vi "Initialization_IPS120_ver1.0.vi"(0 "Magnet Control (IPS 120-10)":T2={"Action"=1, "Standby (s)"=0.0, "Heater on (s)"=300.0, "Sweep Steps "=[], "GPIB ADR"=0, "Change Para?"=FALSE} {"GPIB ADR" items=["None"=0, "25"=25]; "Sweep Steps"."Hold(min)" min=0.0; "Sweep Steps"."Set Rate(T/min)" min=0.001 max=0.5 step=0.001; "Sweep Steps"."Set Point (T)" min=-9.0 max=9.0 step=0.001; "Action" items=["Hold", "To Set Point", "To Zero", "Clamp"]}, 2 "error in":errorcluster, 4 "First run?":bool) -> (1 "Magnet Failed?":bool, 3 "Hold(min)":dbl, 5 "Status":string, 6 "B field Change?":bool, 7 "output cluster":T1={"Com Port"=1, "ISOBUS Address"=1, "GPIB Address"=24, "Communication"=enum."ISOBUS"}, 8 "Target B":string, 9 "Rate":string, 10 "error out":errorcluster)   [LabVIEW 2012]
uses:
  Oxford_itc503/BUSGEN.LLB/OxfordAddress.ctl
panel:
  out "Set point":string
  out "Display":string="+0.00000\r"
  out "Log":string
  # "Current\nField"
  # "T"
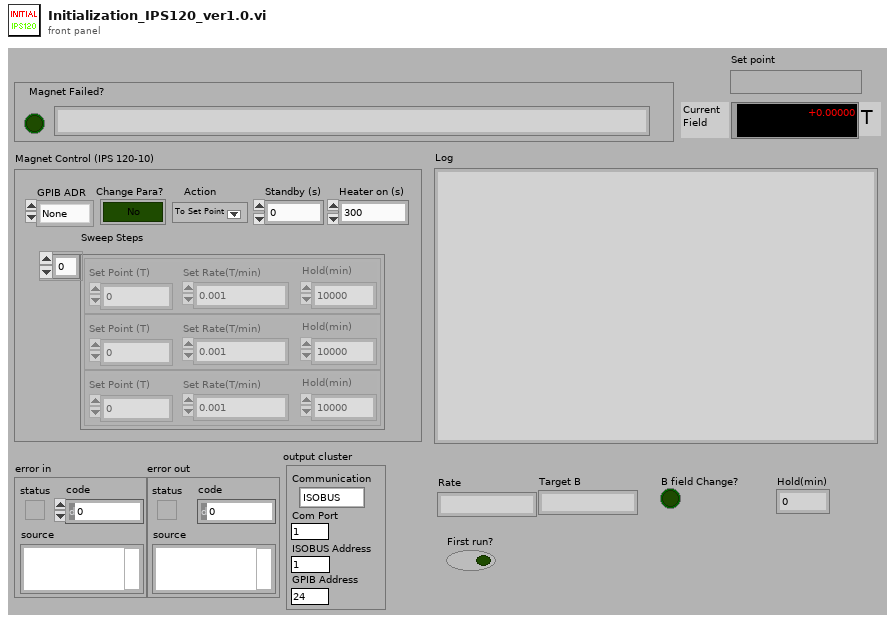
[diagram p1: front panel]
types:
  T1 = cluster{"Com Port":i32, "ISOBUS Address":i32, "GPIB Address":i16, "Communication":enum16{"RS232", "ISOBUS", "GPIB", "Gateway"}}
  T2 = cluster{"Action":u16, "Standby (s)":dbl, "Heater on (s)":dbl, "Sweep Steps ":cluster{"Set Point (T)":dbl, "Set Rate(T/min)":dbl, "Hold(min)":dbl}[], "GPIB ADR":u16, "Change Para?":bool}
  T3 = typedef "OxfordAddress.ctl" = cluster{"Com Port":i32, "ISOBUS Address":i32, "GPIB Address":i16, "Communication":enum16{"RS232", "ISOBUS", "GPIB", "Gateway"}}
  T4 = cluster{"Set Point (T)":dbl, "Set Rate(T/min)":dbl, "Hold(min)":dbl}[]
  T5 = cluster{"Set Point (T)":dbl, "Set Rate(T/min)":dbl, "Hold(min)":dbl}
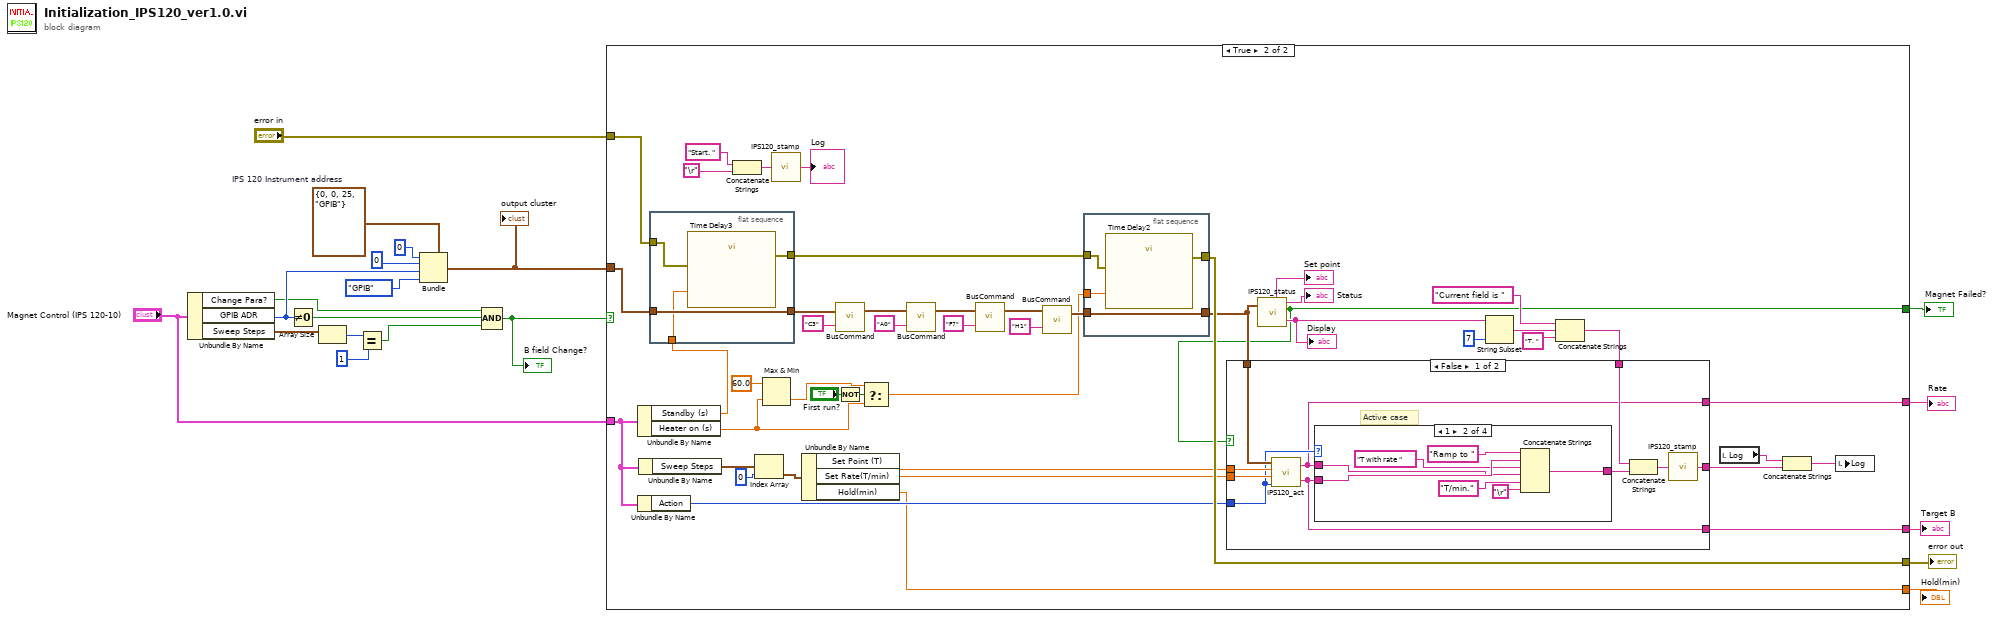
[diagram p0: block diagram]
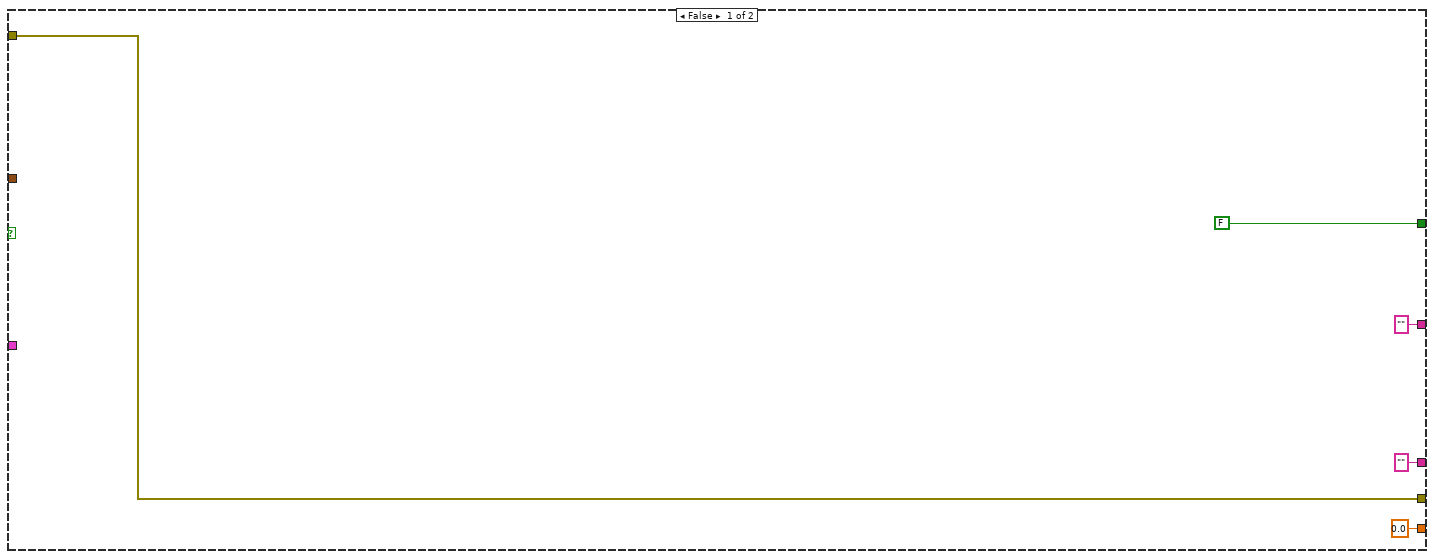
[diagram p2: hidden frame]
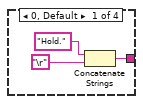
[diagram p3: hidden frame]
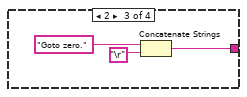
[diagram p4: hidden frame]
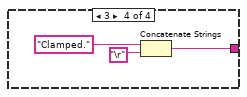
[diagram p5: hidden frame]
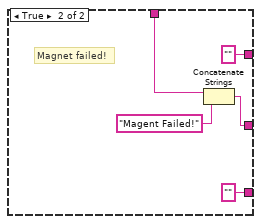
[diagram p6: hidden frame]
diagram:
  w14 = T3 {"Com Port"=0, "ISOBUS Address"=0, "GPIB Address"=25, "Communication"=enum."GPIB"}  # IPS 120 Instrument address
  n1 = Unbundle By Name("Magnet Control (IPS 120-10)") -> ("Change Para?"=w7:bool, "GPIB ADR"=w12:u16, "Sweep Steps"=w11:T4)
  n2 = Not Equal To 0?(x=w12) -> (x != 0?=w6:bool)
  n3 = Array Size(array=w11) -> (size(s)=w10:i32)
  n4 = Equal?(x=w10, y=1) -> (x = y?=w5:bool)
  n5 = Bundle(cluster=w14, "Com Port"=0, "ISOBUS Address"=0, "GPIB Address"=w12, "Communication"=enum16{"RS232", "ISOBUS", "GPIB", "Gateway"}."GPIB") -> (w13:T3)
  "output cluster" <- w13
  n6 = Compound Arithmetic op=AND(w7, w6, w5) -> (w8:bool)
  "B field Change?" <- w8
  n7 = case shown="True" w8 {
    tunnel: "Magnet Control (IPS 120-10)" -> [_ w37]
    tunnel: [w24 w55] -> w19
    tunnel: "error in" -> [w24 w54]
    tunnel: w13 -> [_ w53]
    tunnel: [FALSE w35] -> w4
    tunnel: ["" ("Rate") w34] -> w3
    tunnel: ["" ("Target B") w33] -> w2
    tunnel: [0.0 ("Hold(min)") w32] -> w1
    frame False {
    }
    frame True {
      n8 = Unbundle By Name(w37) -> ("Standby (s)"=w38:dbl, "Heater on (s)"=w28:dbl)
      n9 = Unbundle By Name(w37) -> ("Action"=w36:u16)
      n10 = Unbundle By Name(w37) -> ("Sweep Steps"=w58:T4)
      n11 = flat-sequence {
        tunnel: w53 -> [w107]
        tunnel: [w107] -> w60
        tunnel: w38 -> [w106]
        tunnel: w54 -> [w105]
        tunnel: [w104] -> w59
        frame #0 {
          n12 = call "Time Delay3"("error in (no error)"=w105, "Delay Time (s)"=w106) -> ("error out"=w104:errorcluster)  [unwired: 9 in]
        }
      }
      n13 = Concatenate Strings("Start. " ("Log"), "\r") -> (w70:string)
      n14 = Index Array(array=w58, index=0) -> (element=w56:T5)
      n15 = Max & Min(x=60.0 ("t"), y=w28) -> (min(x,y)=w26:dbl)  [unwired: 1 out]
      n16 = call "IPS120_stamp.vi"("in"=w70) -> ("out"=→"Log":string)
      n17 = Unbundle By Name(w56) -> ("Set Point (T)"=w52:dbl, "Set Rate(T/min)"=w51:dbl, "Hold(min)"=w32:dbl)
      n18 = call "BusCommand.vi"("Command"="C3", "Instrument address (in)"=w60) -> ("Instrument address (out)"=w67:T3)  [unwired: 1 out]
      n19 = Not(x="First run?") -> (.not. x?=w27:bool)
      n20 = Select(t=w26, s=w27, f=w28) -> (s? t:f=w30:dbl)
      n21 = call "BusCommand.vi"("Command"="A0", "Instrument address (in)"=w67) -> ("Instrument address (out)"=w66:T3)  [unwired: 1 out]
      n22 = call "BusCommand.vi"("Command"="F7", "Instrument address (in)"=w66) -> ("Instrument address (out)"=w61:T3)  [unwired: 1 out]
      n23 = call "BusCommand.vi"("Command"="H1", "Instrument address (in)"=w61) -> ("Instrument address (out)"=w62:T3)  [unwired: 1 out]
      n24 = flat-sequence {
        tunnel: w62 -> [w111]
        tunnel: [w111] -> w47
        tunnel: w30 -> [w110]
        tunnel: w59 -> [w109]
        tunnel: [w108] -> w55
        frame #0 {
          n25 = call "Time Delay2"("error in (no error)"=w109, "Delay Time (s)"=w110) -> ("error out"=w108:errorcluster)  [unwired: 9 in]
        }
      }
      n26 = call "IPS120_status.vi"("Address"=w47) -> ("Set point"=→"Set point":string, "Real Field"=w50:string, "Staus"=→"Status":string, "Magnet Failed?"=w35:bool)  [unwired: 1 in, 2 out]
      "Display" <- w50
      n27 = String Subset(string=w50, length (rest)=7 ("length (rest)")) -> (substring=w41:string)  [unwired: 1 in]
      n28 = Concatenate Strings("Current field is " ("string"), w41, "T. " ("string")) -> (w39:string)
      n29 = case shown="False" w35 {
        tunnel: w52 -> [w82 _]
        tunnel: w51 -> [w81 _]
        tunnel: w47 -> [w80 _]
        tunnel: [w79 w101] -> w44
        tunnel: w39 -> [w77 w103]
        tunnel: w36 -> [w75 _]
        tunnel: [w74 "" ("Rate")] -> w34
        tunnel: [w73 "" ("Target B")] -> w33
        frame False {
          # "Active case"
          n30 = call "IPS120_act.vi"("Action"=w75, "Set Rate"=w81, "Set Point"=w82, "Address"=w80) -> ("Target B"=w73:string, "Rate"=w74:string)
          n31 = case shown="1" w75 {
            tunnel: w73 -> [_ w89 _ _]
            tunnel: w74 -> [_ w87 _ _]
            tunnel: [w83 w86 w93 w96] -> w76
            frame 0, Default {
              n32 = Concatenate Strings("Hold." ("Log"), "\r") -> (w83:string)
            }
            frame 1 {
              n33 = Concatenate Strings("Ramp to " ("Log"), w89, "T with rate " ("string"), w87, "T/min." ("format string"), "\r") -> (w86:string)
            }
            frame 2 {
              n34 = Concatenate Strings("Goto zero." ("Log"), "\r") -> (w93:string)
            }
            frame 3 {
              n35 = Concatenate Strings("Clamped." ("Log"), "\r") -> (w96:string)
            }
          }
          n36 = Concatenate Strings(w77, w76) -> (w78:string)
          n37 = call "IPS120_stamp.vi"("in"=w78) -> ("out"=w79:string)
        }
        frame True {
          # "Magnet failed!"
          n38 = Concatenate Strings(w103, "Magent Failed!" ("string")) -> (w101:string)
        }
      }
      n39 = local read "Log"() -> (w43:string)
      n40 = Concatenate Strings(w43, w44) -> (w45:string)
      n41 = local write "Log"(w45) -> ()
    }
  }
  "error out" <- w19
  "Magnet Failed?" <- w4
  "Rate" <- w3
  "Target B" <- w2
  "Hold(min)" <- w1
